vi "_script_parse_arg.vi"(11 "QD Text":string) -> (3 "args":string[](array[string]))   [LabVIEW 2019, in "Script.lvlib"]
doc: "Parses the Quick Drop Textbox arguments by whitespace.\n\nCreated by: Ryan Pacini"
uses:
  Script.lvlib
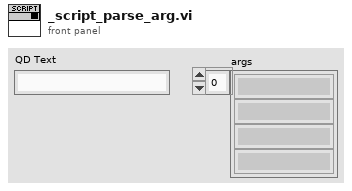
[diagram p1: front panel]
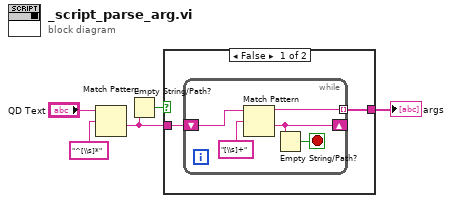
[diagram p0: block diagram]
diagram:
  n1 = Match Pattern(string="QD Text", regular expression="^[\\s]*") -> (after substring=w1:string)  [unwired: 1 in, 3 out]
  n2 = Empty String/Path?(string/path=w1) -> (empty?=w4:bool)
  n3 = case shown="False" w4 {
    tunnel: [w7 _] -> w5
    tunnel: w1 -> [w6 _]
    frame False {
      n4 = while {
        tunnel: [w12] -> w7 mode=indexing
        shift-right: [w8] -> _
        shift-left: w6 -> [w10]
        stop <- w9 stop-if-true
        n5 = Match Pattern(string=w10, regular expression="[\\s]+") -> (before substring=w12:string, after substring=w8:string)  [unwired: 1 in, 2 out]
        n6 = Empty String/Path?(string/path=w8) -> (empty?=w9:bool)
      }
    }
    frame True {
    }
  }
  "args" <- w5
